vi "SwitchesMirrors Data.vi"() -> (0 "LaserVideo Data":T1={"Configuration"={"Relay VISA Session"="COM1", "Switches"={"Laser"=FALSE, "Video"=FALSE}, "Delays (ms)"={"Laser"=500, "Video"=1500}}, "Refnums"={"Instrument Status"=refnum, "Laser"=refnum, "Video"=refnum, "Relay VISA"=refnum}, "Initialize"={"Update Refnums"=FALSE, "Connect"=FALSE, "Set Configuration"=FALSE}})   [LabVIEW 2014]
uses:
  SwitchesMirrors Data.ctl
  SwitchesMirrors Config.ctl
  SwitchesMirrors Status.ctl
  SwitchesMirrors Refnum.ctl
  support/Instrument Status.ctl
  SwitchesMirrors Initialize.ctl
panel:
  # "LICENSED MATERIALS – PROPERTY OF IBM\nCopyright IBM Corp. 2016,\nALL RIGHTS RESERVED"
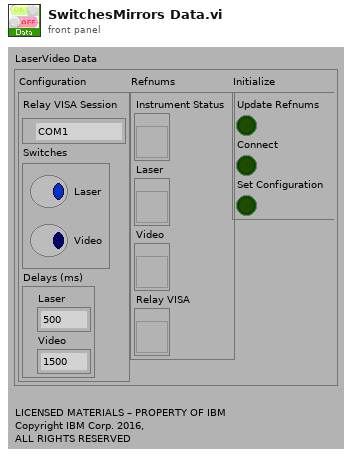
[diagram p1: front panel]
types:
  T1 = typedef "SwitchesMirrors Data.ctl" = cluster{"Configuration":T2, "Refnums":T4, "Initialize":T5}
  T2 = typedef "SwitchesMirrors Config.ctl" = cluster{"Relay VISA Session":refnum<visa-resource-name>, "Switches":T3, "Delays (ms)":cluster{"Laser":u32, "Video":u32}}
  T3 = typedef "SwitchesMirrors Status.ctl" = cluster{"Laser":bool, "Video":bool}
  T4 = typedef "SwitchesMirrors Refnum.ctl" = cluster{"Instrument Status":refnum<vi>, "Laser":refnum<vi>, "Video":refnum<vi>, "Relay VISA":refnum<vi>}
  T5 = typedef "SwitchesMirrors Initialize.ctl" = cluster{"Update Refnums":bool, "Connect":bool, "Set Configuration":bool}
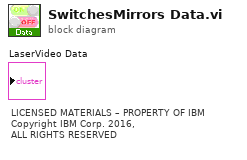
[diagram p0: block diagram]
diagram:
  # "LICENSED MATERIALS – PROPERTY OF IBM\nCopyright IBM Corp. 2016,\nALL RIGHTS RESERVED"
